vi "WPI_I2CRefNum Registry Get.vi"(8 "error in (no error)":errorcluster, 10 "refnum name":string="My I2C RefNum") -> (0 "error out":errorcluster, 3 "I2CDevRef":T1={"DevStatus"={"status"=FALSE, "code"=0, "source"=""}, "Device Address"=0, "Handle"=0, "I2C Bus"=enum."Invalid"} {"Device Address" format="%.0x"})   [LabVIEW 2017]
doc: "Gets the reference you specify. You first must set the reference with the RefNum Registry Set VI."
uses:
  <vilib>/Rock Robotics/WPI/I2C/WPI_I2CDevRef.ctl
  <vilib>/Rock Robotics/SystemInterfaces/i2clib/i2c_bus.ctl
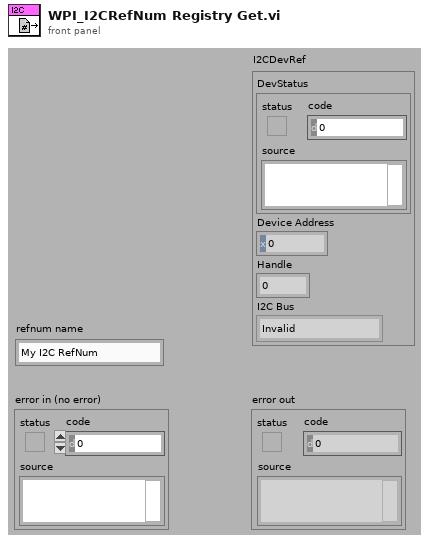
[diagram p1: front panel]
types:
  T1 = typedef "WPI_I2CDevRef.ctl" = cluster{"DevStatus":errorcluster, "Device Address":u8, "Handle":i32, "I2C Bus":T2}
  T2 = typedef "i2c_bus.ctl" = enum16{"I2C On-Board", "I2C MXP", "Invalid"}
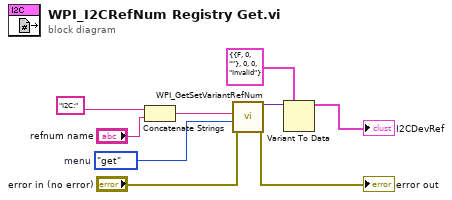
[diagram p0: block diagram]
diagram:
  w2 = enum16{"set", "get", "delete"}."get"  # menu
  n1 = Concatenate Strings("I2C:", "refnum name") -> (w9:string)
  n2 = call <vilib>:"WPI_GetSetVariantRefNum.vi"("error in (no error)"="error in (no error)", "Operation"=w2, "refnum name"=w9) -> ("error out"=→"error out":errorcluster, "DevRef"=w7:variant)  [unwired: 6 in, 1 out]
  n3 = Variant To Data(type=T1 {"DevStatus"={"status"=FALSE, "code"=0, "source"=""}, "Device Address"=0, "Handle"=0, "I2C Bus"=enum."Invalid"} ("I2CDevRef"), Variant=w7) -> (data=→"I2CDevRef":T1)  [unwired: 1 in, 1 out]
